vi "APF for CF.vi"(7 "Input Signal Sample (q)":dbl, 9 "C":dbl) -> (1 "Output Signal Sample (r)":dbl)   [LabVIEW 2011]
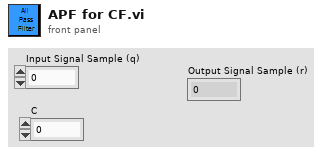
[diagram p1: front panel]
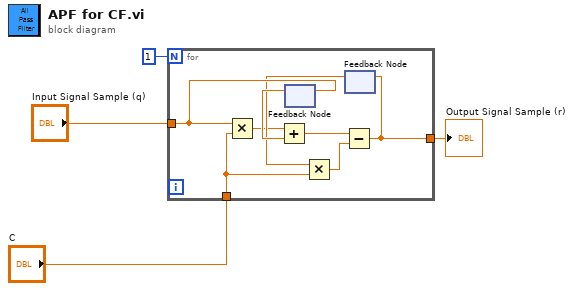
[diagram p0: block diagram]
diagram:
  n1 = for {
    N: 1 -> [_]
    tunnel: [w9] -> w3
    tunnel: "Input Signal Sample (q)" -> [w11]
    tunnel: "C" -> [w5]
    n2 = Multiply(x=w11, y=w5) -> (x*y=w6:dbl)
    n3 = feedback #1() -> (w12:dbl)  [unwired: 1 in]
    n4 = Add(x=w6, y=w12) -> (x+y=w8:dbl)
    n5 = feedback-in #1(w11) -> ()
    n6 = feedback #2() -> (w10:dbl)  [unwired: 1 in]
    n7 = Multiply(x=w10, y=w5) -> (x*y=w7:dbl)
    n8 = Subtract(x=w8, y=w7) -> (x-y=w9:dbl)
    n9 = feedback-in #2(w9) -> ()
  }
  "Output Signal Sample (r)" <- w3
